vi "hasNext.vi"(8 "error in (no error)":errorcluster, 11 "NameIterator in":refnum<class "NameIterator.lvclass">) -> (0 "error out":errorcluster, 2 "hasNext?":bool, 3 "NameIterator out":refnum<class "NameIterator.lvclass">)   [LabVIEW 2018, in "NameIterator.lvclass"]
uses:
  NameIterator.lvclass
  NameIterator.lvclass/NameIterator.ctl
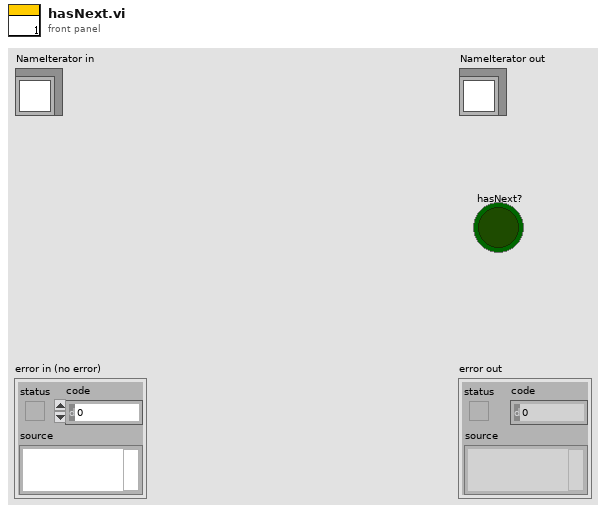
[diagram p1: front panel]
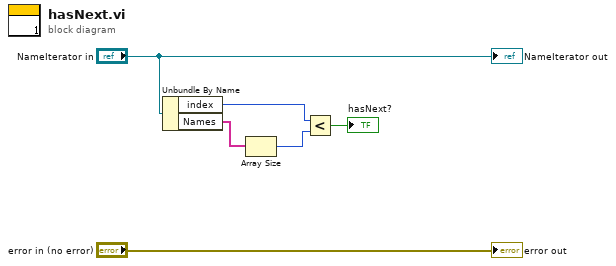
[diagram p0: block diagram]
diagram:
  n1 = Unbundle By Name("NameIterator in") -> ("index"=w4:i32, "Names"=w1:string[])
  n2 = Array Size(array=w1) -> (size(s)=w3:i32)
  n3 = Less?(x=w4, y=w3) -> (x < y?=→"hasNext?":bool)
  "error out" <- "error in (no error)"
  "NameIterator out" <- "NameIterator in"
